vi "Open.vi"(8 "error in":errorcluster, 9 "parameters":variant, 10 "file path":path, 11 "repository in":refnum<class "CustomDeviceRepo.lvclass">) -> (0 "error out":errorcluster, 2 "invalid?":bool, 3 "repository out":refnum<class "CustomDeviceRepo.lvclass">)   [LabVIEW 2015, in "CustomDeviceRepo.lvclass"]
doc: "Loads the saved information of the repo. It could load multiple files at the same time. An option to add file versioning could be included in the files, and the code to manage changes would be in this VI."
uses:
  CustomDeviceRepo.lvclass
  CustomDeviceRepo.lvclass/CustomDeviceRepo.ctl
  Configuration Tool.lvlib
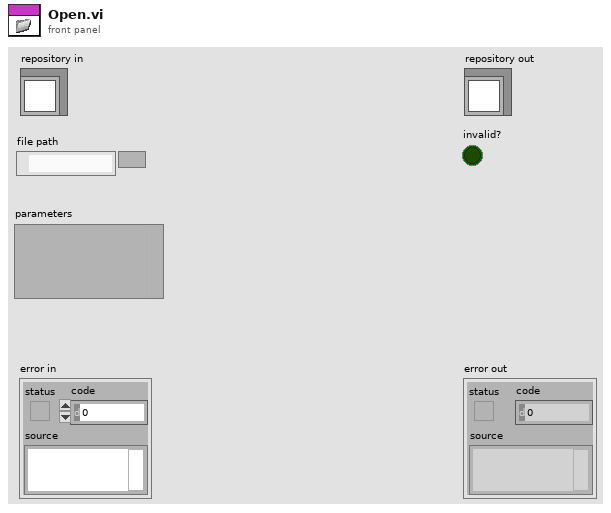
[diagram p1: front panel]
types:
  T1 = typedef "Main Custom Device Properties.ctl" = cluster{"CD Name":string, "Version":string, "Max Occurrences":i32, "Device Type":enum16{"Asynchronous", "Inline HW Interface", "Inline Model Interface", "Inline Timing and Sync", "Asynchronous Timing and Sync"}, "Main Page GUID":string}
  T2 = typedef "Initialization VI Properties.ctl" = cluster{"Execution":T3, "Path":T4, "Type":enum16{"Action", "VI"}, "Position":enum16{"centered", "mouse pointer"}}
  T3 = typedef "Configuration Tool.lvlib/Execution Types.ctl" = enum16{"silent", "modal", "floating", "default"}
  T4 = typedef "Configuration Tool.lvlib/Path Cluster.ctl" = cluster{"Path":path, "Path Type":enum16{"Absolute", "To Base", "To Common Doc Dir", "To Application Data Dir"}}
  T5 = typedef "Timing Source Properties.ctl" = cluster{"Has Timing Source Capability":bool, "Source Distribution":T6}
  T6 = typedef "Configuration Tool.lvlib/Source Distribution for TimingSource.ctl" = cluster{"Supported Target":T7, "Source":T4, "Real Time System Destination":string, "Version":string}[]
  T7 = typedef "Configuration Tool.lvlib/Target.ctl" = enum16{"All", "Pharlap", "VxWorks", "Windows", "Linux_32_ARM", "Linux_x64", "PharlapWindows", "PharlapVxWorks", "VxWorksWindows"}
  T8 = typedef "Configuration Tool.lvlib/Custom Device VI.ctl" = cluster{"Source Distribution":cluster{"Source Distribution - Sources":T9}, "Source":T4, "Real Time System Destination":string}
  T9 = typedef "Configuration Tool.lvlib/Source Distribution for Custom Device VI.ctl" = cluster{"Source":T4, "Real Time System Destination":string, "Supported Target":T7}[]
  T10 = typedef "Configuration Tool.lvlib/Page.ctl" = cluster{"Name":string, "Disallow Renaming":bool, "Delete Protection":bool, "Exlcude from Alphabetical order":bool, "Allow Multi-Selection":bool, "GUID":string, "Parent GUIDs":string[], "Glyph":T4, "Inactive Glyph":T4, "Broken Glyph":T4, "Item to Launch":T4, "Action VI On Delete":T4, "Action VI On Load":T4, "Action VI On Paste":T4, "Action VI On Target Type Change":T4, "Action VI On Delete Request":T4, "Action VI On Compile":T4, "Additional Information":string, "Run Time Menu":T11[], "Button List":T13[], "Action VI On System Shutdown":T4, "Action VI On Save":T4, "Action VI On Download":T4, "Copy":enum16{"copy", "disabled"}, "Paste":enum16{"Create", "CreatIfNotExists_GUID", "CreatIfNotExists_Name", "Replace", "Dialog"}, "Help":T15}
  T11 = typedef "Configuration Tool.lvlib/Menu Item.ctl" = cluster{"GUID":string, "Execution":T3, "MinNrOfChilds":u32, "Name":string, "Item to Launch":T4, "Dependency":T12, "Custom Population":T4, "Menu Item Type":enum16{"Action", "VI", "Separator", "Custom"}, "Behavior":enum16{"Nothing", "Open Front Panel"}, "Position":enum16{"Centered", "Mouse Pointer"}}
  T12 = typedef "Configuration Tool.lvlib/Dependency three item small.ctl" = cluster{"File Path Control":path, "Path Type":enum16{"Absolute", "To Base", "To Common Doc Dir", "To Application Data Dir"}, "Behavior":enum16{"Static", "Dynamic"}}
  T13 = typedef "Configuration Tool.lvlib/Button.ctl" = cluster{"ID":string, "Glyph":T4, "Button Type":T14, "Referenced GUID":string, "Button Text":string, "Caption":string, "Tip Strip":string, "Documentation":string, "Dependency":T12}
  T14 = typedef "Configuration Tool.lvlib/Button Type.ctl" = enum16{"Action", "Dialog", "Page", "Notification", "Separator"}
  T15 = typedef "Configuration Tool.lvlib/help.ctl" = cluster{"Item to Launch":T4, "Section":string, "File Type":enum16{"chm", "other"}}
  T16 = enum16{"Create", "CreatIfNotExists_GUID", "CreatIfNotExists_Name", "Replace", "Dialog"}
  T17 = cluster{"Action VI On Delete":T4, "Action VI On Load":T4, "Action VI On Paste":T4, "Action VI On Target Type Change":T4, "Action VI On Delete Request":T4, "Action VI On Compile":T4, "Action VI On System Shutdown":T4, "Action VI On Save":T4, "Action VI On Download":T4}
  T18 = cluster{"Name":string, "Disallow Renaming":bool, "Delete Protection":bool, "Exlcude from Alphabetical order":bool, "Allow Multi-Selection":bool, "GUID":string, "Parent GUIDs":string[], "Glyph":T4, "Inactive Glyph":T4, "Broken Glyph":T4, "Item to Launch":T4, "Additional Information":string, "Copy":enum16{"copy", "disabled"}, "Paste":enum16{"Create", "CreatIfNotExists_GUID", "CreatIfNotExists_Name", "Replace", "Dialog"}, "Help":T15}
  T19 = cluster{cluster{"Name":string, "Disallow Renaming":bool, "Delete Protection":bool, "Exlcude from Alphabetical order":bool, "Allow Multi-Selection":bool, "GUID":string, "Parent GUIDs":string[], "Glyph":T4, "Inactive Glyph":T4, "Broken Glyph":T4, "Item to Launch":T4, "Additional Information":string, "Copy":enum16{"copy", "disabled"}, "Paste":enum16{"Create", "CreatIfNotExists_GUID", "CreatIfNotExists_Name", "Replace", "Dialog"}, "Help":T15}, cluster{"Action VI On Delete":T4, "Action VI On Load":T4, "Action VI On Paste":T4, "Action VI On Target Type Change":T4, "Action VI On Delete Request":T4, "Action VI On Compile":T4, "Action VI On System Shutdown":T4, "Action VI On Save":T4, "Action VI On Download":T4}, "Button List":T13[], "Run Time Menu":T11[]}
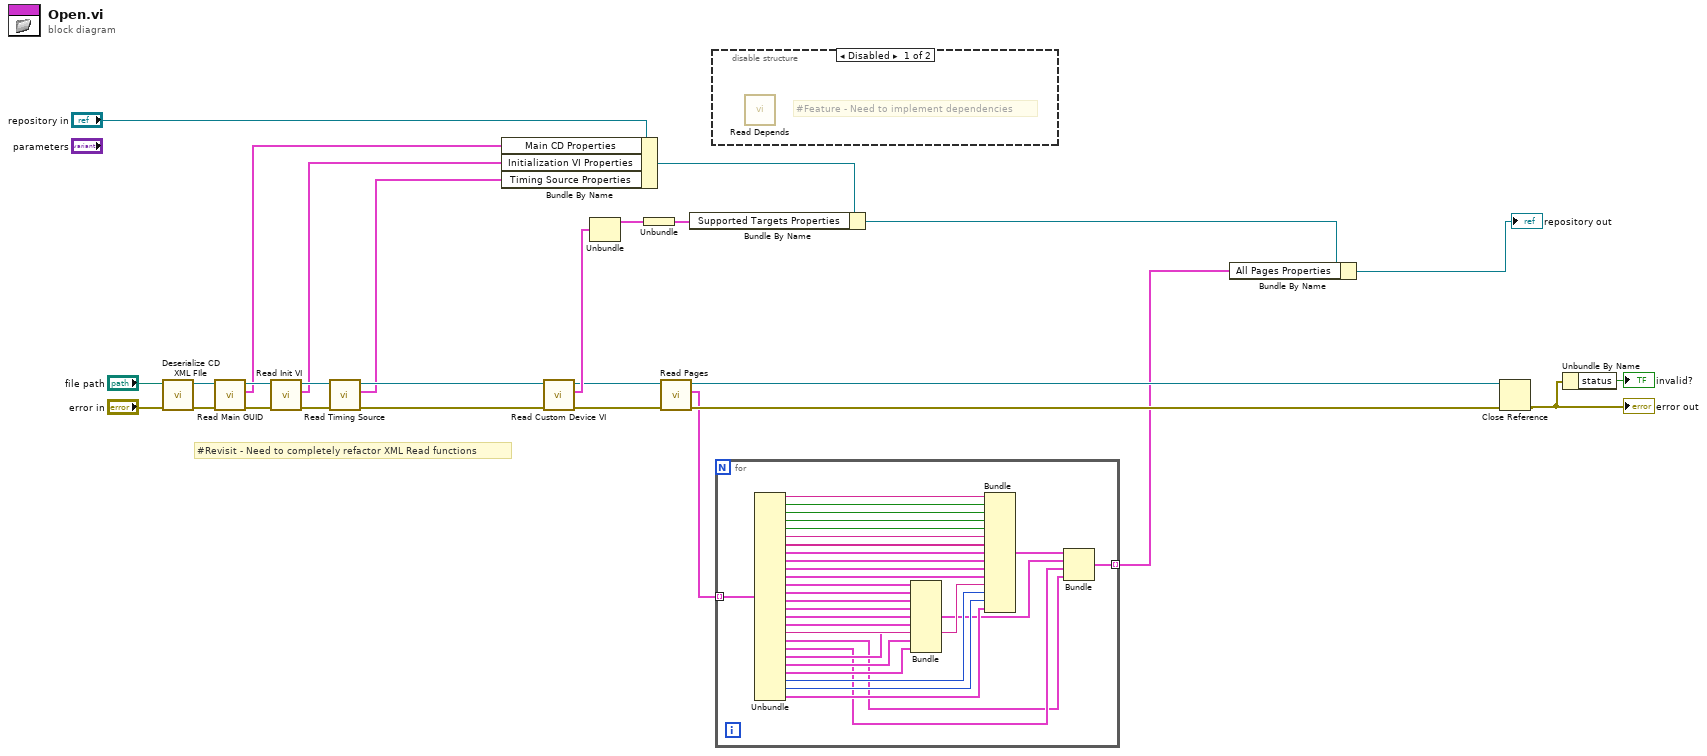
[diagram p0: block diagram]
diagram:
  # "#Revisit - Need to completely refactor XML Read functions"
  n1 = call "Deserialize CD XML FIle.vi"("Error In"="error in", "XML Path"="file path") -> ("Error Out"=w26:errorcluster, "Custom Device .NET Ref Out"=w25:refnum<k24>)  [unwired: 8 in]
  n2 = call "Read Main GUID.vi"("Error In"=w26, "Custom Device .NET Ref In"=w25) -> ("Error out"=w19:errorcluster, "Main CD Properties"=w3:T1, "Custom Device .NET Ref Out"=w20:refnum<k24>)  [unwired: 7 in]
  n3 = call "Read Init VI.vi"("Error In"=w19, "Custom Device .NET Ref In"=w20) -> ("Error Out"=w18:errorcluster, "Initialization VI Properties"=w2:T2, "Custom Device .NET Ref Out"=w17:refnum<k24>)  [unwired: 7 in]
  n4 = call "Read Timing Source.vi"("Error In"=w18, "Custom Device .NET Ref In"=w17) -> ("Error Out"=w16:errorcluster, "Timing Source Properties"=w1:T5, "Custom Device .NET Ref Out"=w15:refnum<k24>)  [unwired: 7 in]
  n5 = Bundle By Name(cluster="repository in", "Main CD Properties"=w3, "Initialization VI Properties"=w2, "Timing Source Properties"=w1) -> (w21:refnum<class "CustomDeviceRepo.lvclass">)
  n6 = call "Read Custom Device VI.vi"("error in"=w16, "Custom Device reference in"=w15) -> ("error out"=w10:errorcluster, "Custom Device VI"=w14:T8, "Custom Device reference out"=w11:refnum<k24>)  [unwired: 7 in]
  n7 = Unbundle(w14) -> ("Source Distribution"=w13:cluster{"Source Distribution - Sources":T9})  [unwired: 2 out]
  n8 = Unbundle(w13) -> ("Source Distribution - Sources"=w12:T9)
  n9 = call "Read Pages.vi"("error in"=w10, "Custom Device reference in"=w11) -> ("error out"=w8:errorcluster, "Pages"=w7:T10[], "Custom Device reference out"=w9:refnum<k24>)  [unwired: 7 in]
  n10 = Bundle By Name(cluster=w21, "Supported Targets Properties"=w12) -> (w6:refnum<class "CustomDeviceRepo.lvclass">)
  n11 = disable-structure shown="Disabled" {
    frame Disabled {
      # "#Feature - Need to implement dependencies"
      n12 = call "Read Depends.vi"() -> ()  [unwired: 9 in, 3 out]
    }
    frame Enabled {
    }
  }
  n13 = for {
    tunnel: w7 -> [w58] mode=indexing
    tunnel: [w32] -> w4 mode=indexing
    n14 = Unbundle(w58) -> ("Name"=w57:string, "Disallow Renaming"=w56:bool, "Delete Protection"=w47:bool, "Exlcude from Alphabetical order"=w48:bool, "Allow Multi-Selection"=w49:bool, "GUID"=w50:string, "Parent GUIDs"=w55:string[], "Glyph"=w51:T4, "Inactive Glyph"=w52:T4, "Broken Glyph"=w53:T4, "Item to Launch"=w54:T4, "Action VI On Delete"=w42:T4, "Action VI On Load"=w41:T4, "Action VI On Paste"=w40:T4, "Action VI On Target Type Change"=w39:T4, "Action VI On Delete Request"=w38:T4, "Action VI On Compile"=w37:T4, "Additional Information"=w46:string, "Run Time Menu"=w29:T11[], "Button List"=w30:T13[], "Action VI On System Shutdown"=w36:T4, "Action VI On Save"=w35:T4, "Action VI On Download"=w34:T4, "Copy"=w45:enum16{"copy", "disabled"}, "Paste"=w44:T16, "Help"=w43:T15)
    n15 = Bundle("Action VI On Delete"=w42, "Action VI On Load"=w41, "Action VI On Paste"=w40, "Action VI On Target Type Change"=w39, "Action VI On Delete Request"=w38, "Action VI On Compile"=w37, "Action VI On System Shutdown"=w36, "Action VI On Save"=w35, "Action VI On Download"=w34) -> (w31:T17)  [unwired: 1 in]
    n16 = Bundle("Name"=w57, "Disallow Renaming"=w56, "Delete Protection"=w47, "Exlcude from Alphabetical order"=w48, "Allow Multi-Selection"=w49, "GUID"=w50, "Parent GUIDs"=w55, "Glyph"=w51, "Inactive Glyph"=w52, "Broken Glyph"=w53, "Item to Launch"=w54, "Additional Information"=w46, "Copy"=w45, "Paste"=w44, "Help"=w43) -> (w33:T18)  [unwired: 1 in]
    n17 = Bundle(w33, w31, "Button List"=w30, "Run Time Menu"=w29) -> (w32:T19)  [unwired: 1 in]
  }
  n18 = Bundle By Name(cluster=w6, "All Pages Properties"=w4) -> (→"repository out":refnum<class "CustomDeviceRepo.lvclass">)
  n19 = Close Reference(reference=w9, error in (no error)=w8) -> (error out=w22:errorcluster)
  "error out" <- w22
  n20 = Unbundle By Name(w22) -> ("status"=→"invalid?":bool)
